vi "7HP.vi"() -> (0 "DAQ Error":errorcluster)   [LabVIEW 2017]
doc: "Use this plug-in with the Nathan 7609 data acquisition system"
uses:
  7HP/ctls/Cmd (USB).ctl
  Globals/Meas_global.vi
  Globals/Extra_Commands_Global.vi
  Globals/Dynamic_call_global.ph.vi
  Globals/Trav_pos_global.vi
panel:
  # "Do not close this window between blocks"
  # "PN 18/10/2017"
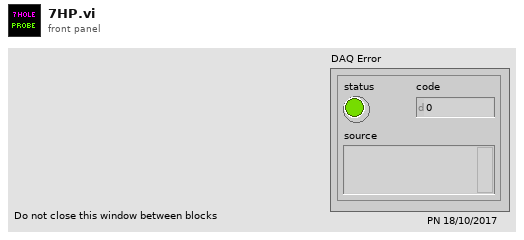
[diagram p1: front panel]
types:
  T1 = typedef "Analysis_info_cluster.ctl" = cluster{"Colour":u32, "Inst type":T2, "Inst name":string, "Symbol":string, "Code name":string, "Extra Info":string, "Inst Array":T3, "Extra Titles":string[], "Extra Values":string[], "U":dbl, "u^2":dbl, "u^3":dbl, "u^4":dbl, "Skew_u":dbl, "Kurt_u":dbl, "Sd Error in Mean":dbl, "% u'/U":dbl, "X":dbl, "Y":dbl, "Z":dbl, "Timescale integral Estimate":dbl, "Sd Error in Variance":dbl, "Calib File":path, "Calib Constants":dbl[], "Output Position":bool, "Full Stats":bool, "Av Sampling Rate":dbl, "Av No of Samples":dbl, "Total Meas Time (s)":dbl, "ADAM Ch Name":string, "Max value":dbl, "Min value":dbl, "Req Sample Rate Hz":dbl, "Sync Delay Time (s)":dbl, "Ch No":i16, "Device ID":string, "Use Latest Calib":bool, "Port":string}
  T2 = typedef "Inst_type.ctl" = enum16{"Propeller anemometer", "Raw voltage", "Pressure Transducer", "Pitot-static tube", "Preston tube", "Hot wire", "Cross wire 1", "Cross wire 2", "Generic Linear", "Generic Polynomial", "Generic BackPoly", "Fast FID", "Thermocouple", "Cold wire", "Pulsed Wire", "LDA Vel", "LDA Tran time", "LDA Arr time", "Microphone"}
  T3 = typedef "Instrument_Array.ctl" = enum16{"PWA", "LDA", "Analogue"}
  T4 = typedef "Traverse_cluster.ctl" = cluster{"Start X":sgl, "Start Y":sgl, "Start Z":sgl, "End X":sgl, "End Y":sgl, "End Z":sgl, "No. of pts.":i32, "Spacing":T5, "Filename":path, "Tunnel Speed":dbl, "Averaging time (min)":dbl, "Extra Commands":string, "Carrier_1 Q (l/min)":dbl, "Carrier_2 Q (l/min)":dbl, "Trace Gas Concentration (%)":dbl, "Specific Arguments":string, "Comments":string, "Row No":i32, "Row Type Selector":T6, "Completion time":string, "Row Duration (mins)":dbl, "No. of Valid pts.":i32, "Meas Setup File":string}
  T5 = typedef "Spacing.ctl" = enum16{"Linear", "Log", "Gauss", "Specified", "N/A"}
  T6 = typedef "Multi_run_mode.ctl" = enum16{"Move Traverse Only", "Set Tunnel Speed Only", "Set Source Only", "Set Measurement Conditions", "Single Measurement", "Vertical Profile", "Lateral Profile", "Longitudinal Profile", "Explore Volume", "Multi-Axis Profile", "Auto Calibrate", "Meas Fast FID Bkgnd", "Check Beam Power", "Scanning Valve Measurement", "Run VI Named:", "Set ADAM Ch", "Wait (minutes)", "Send Message", "Synchronize With:", "Fall Back to this Row", "Turn Off Row Repeating", "Blank Row", "Traverse 3D Volume"}
  T7 = typedef "Trigger_Mode.ctl" = enum16{"Free Running", "Start on Trigger", "Trigger Every Block", "Trigger Every Sample"}
  T8 = typedef "Cmd (USB).ctl" = string
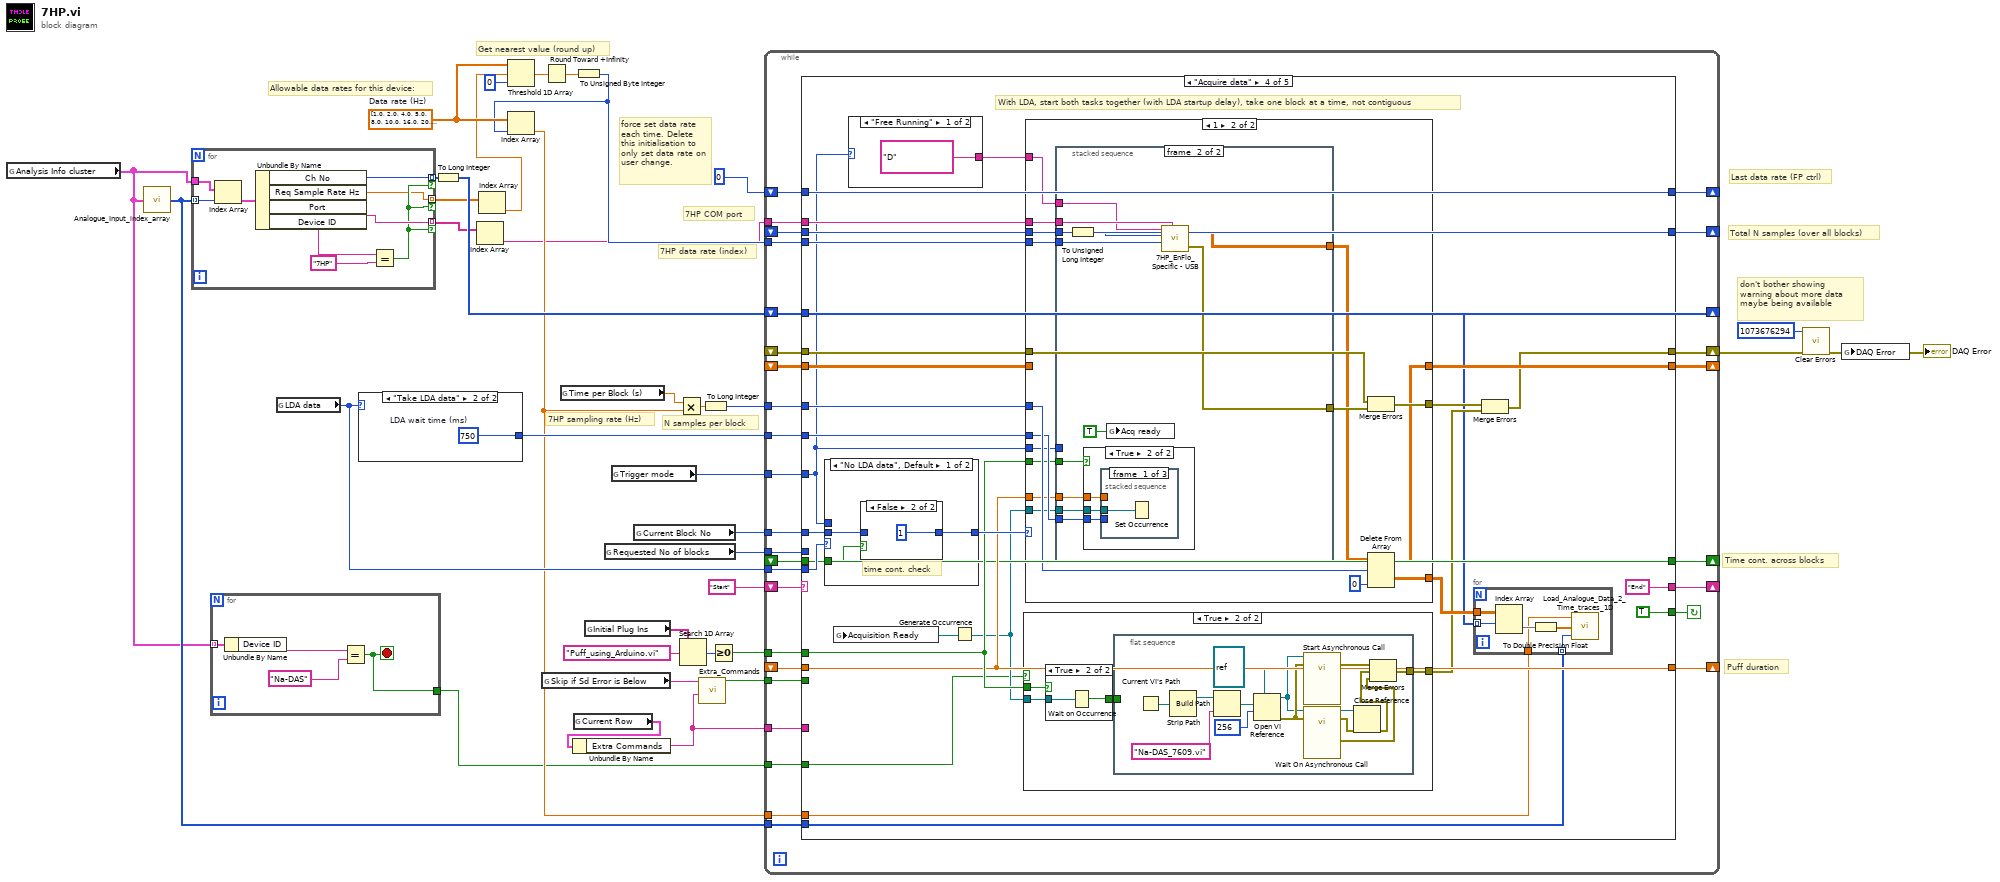
[diagram p0: block diagram]
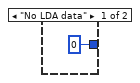
[diagram p2: hidden frame]
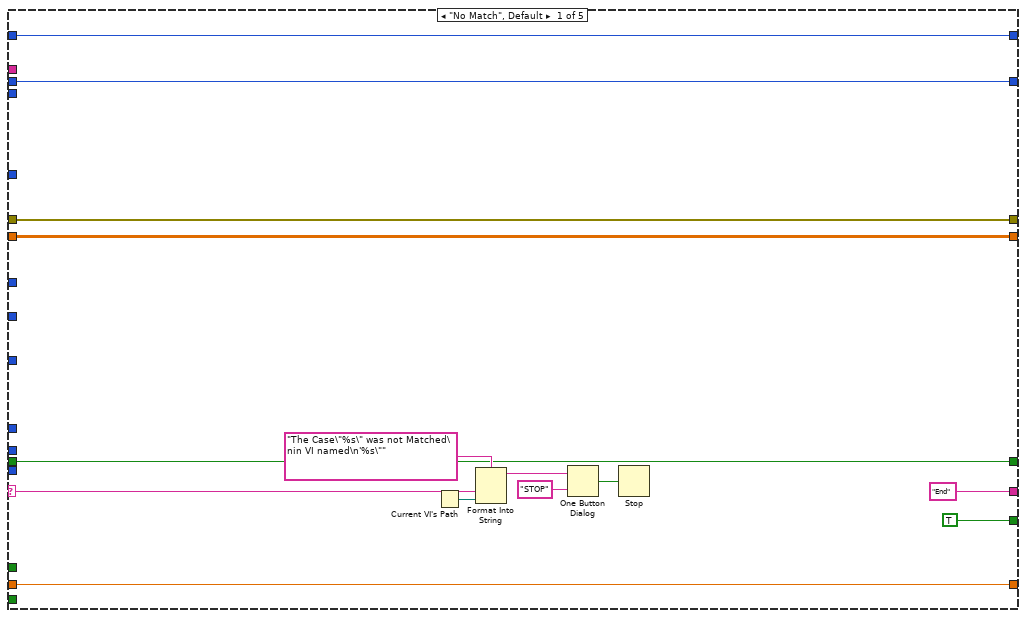
[diagram p3: hidden frame]
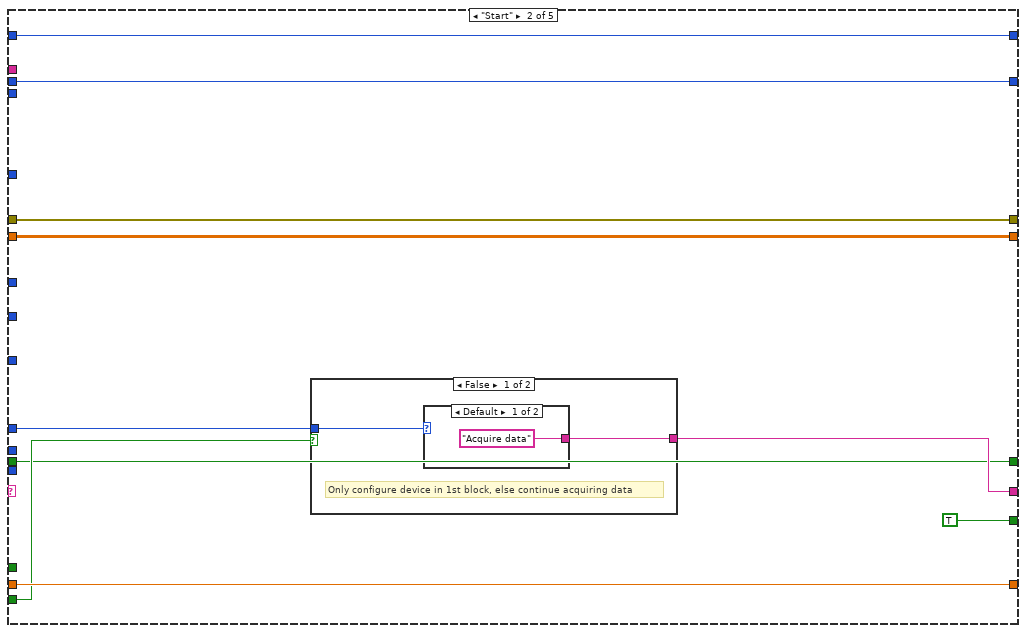
[diagram p4: hidden frame]
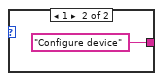
[diagram p5: hidden frame]
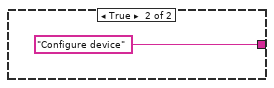
[diagram p6: hidden frame]
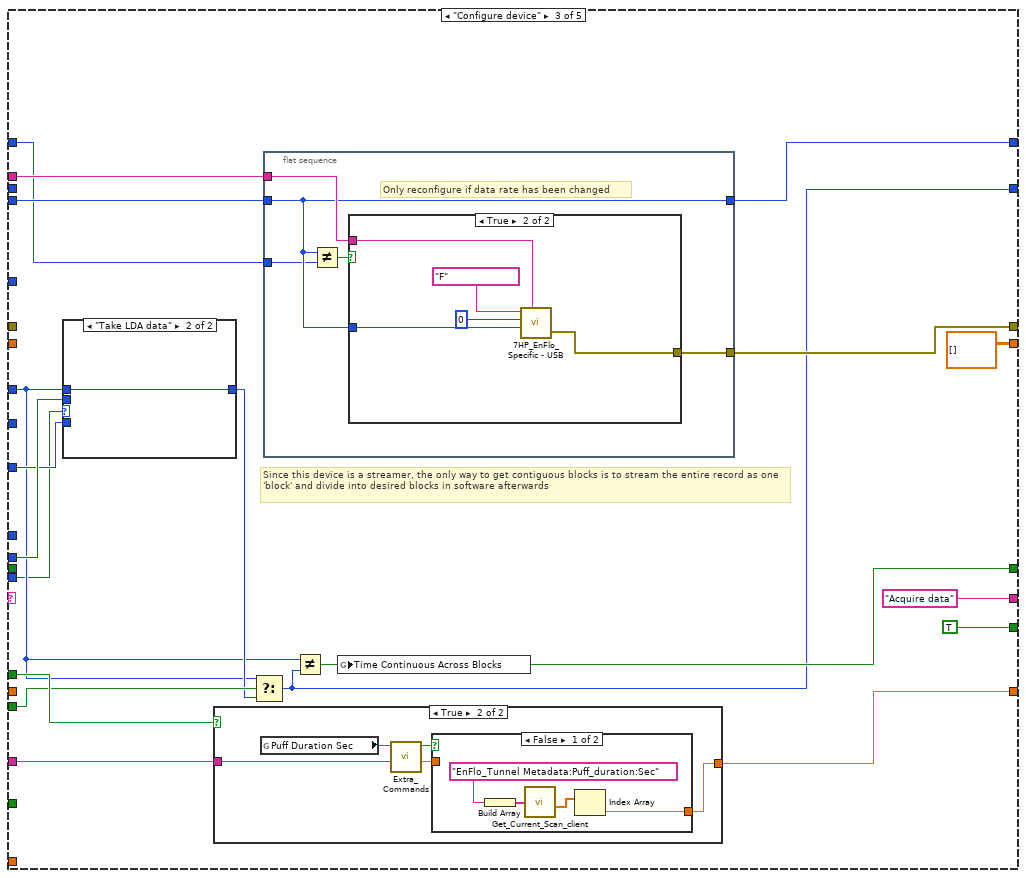
[diagram p7: hidden frame]
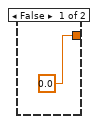
[diagram p8: hidden frame]
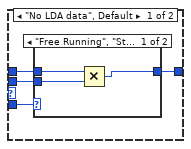
[diagram p10: hidden frame]
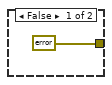
[diagram p12: hidden frame]
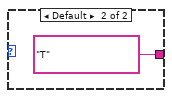
[diagram p13: hidden frame]
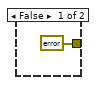
[diagram p14: hidden frame]
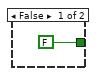
[diagram p15: hidden frame]
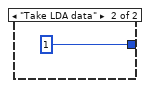
[diagram p17: hidden frame]
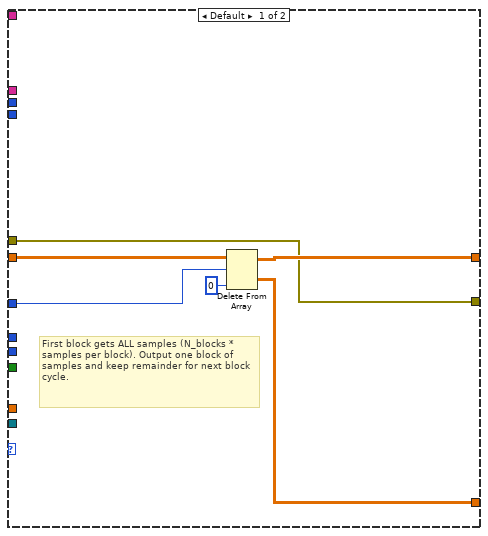
[diagram p18: hidden frame]
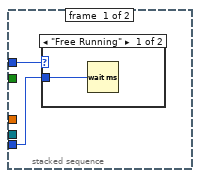
[diagram p19: hidden frame]
diagram:
  w16 = dbl[] [1.0, 2.0, 4.0, 5.0, 8.0, 10.0, 16.0, 20.0, 25.0, 32.0, 40.0, 50.0, 64.0, 80.0, 100.0, 125.0, 160.0, 200.0, 250.0, 320.0, 400.0, 500.0, 625.0, 800.0, 1000.0]  # Data rate (Hz)
  # "N samples per block"
  # "7HP sampling rate (Hz)"
  # "7HP COM port"
  # "7HP data rate (index)"
  # "Allowable data rates for this device:"
  # "Get nearest value (round up)"
  # "force set data rate each time. Delete this initialisation to only set data rate on user change."
  # "Last data rate (FP ctrl)"
  # "Total N samples (over all blocks)"
  # "don't bother showing warning about more data maybe being available"
  # "Time cont. across blocks"
  # "Puff duration"
  n1 = global read "Meas_global.vi" "Analysis Info cluster"() -> (w2:T1[])
  n2 = call "Analogue_Input_index_array.vi"("Analysis Info cluster"=w2) -> ("Array"=w9:i32[])
  n3 = for {
    tunnel: [w45] -> w14 mode=indexing if=w38
    tunnel: [w37] -> w3 mode=indexing if=w38
    tunnel: w2 -> [w44]
    tunnel: w9 -> [w43] mode=indexing
    tunnel: [w41] -> w6 mode=indexing if=w38
    n4 = Index Array(array=w44, index=w43) -> (element=w42:T1)
    n5 = Unbundle By Name(w42) -> ("Ch No"=w45:i16, "Req Sample Rate Hz"=w37:dbl, "Port"=w41:string, "Device ID"=w40:string)
    n6 = Equal?(x=w40, y="7HP" ("Device ID")) -> (x = y?=w38:bool)
  }
  n7 = for {
    tunnel: w2 -> [w47] mode=indexing
    tunnel: [w46] -> w1
    stop <- w46 stop-if-true
    n8 = Unbundle By Name(w47) -> ("Device ID"=w49:string)
    n9 = Equal?(x=w49, y="Na-DAS" ("Device ID")) -> (x = y?=w46:bool)
  }
  n10 = global read "Meas_global.vi" "LDA data"() -> (w33:enum16{"No LDA data", "Take LDA data"})
  n11 = case shown="\"Take LDA data\"" w33 {
    tunnel: [u32 0 ("LDA wait time (ms)") w51] -> w28
    frame "No LDA data" {
    }
    frame "Take LDA data" {
      w51 = u32 750  # LDA wait time (ms)
    }
  }
  n12 = To Long Integer(number=w14) -> (32bit integer=w13:i32[])
  n13 = Index Array(array=w6) -> (element=w5:string)  [unwired: 1 in]
  n14 = Index Array(array=w3) -> (element=w4:dbl)  [unwired: 1 in]
  n15 = Threshold 1D Array(1:0 ("start index (0)"), 2:w4, 3:w16) -> (0:w17:dbl)
  n16 = global read "Extra_Commands_Global.vi" "Skip if Sd Error is Below"() -> (w25:string)
  n17 = Round Toward +Infinity(x=w17) -> (ceil(x): smallest int >= x=w15:dbl)
  n18 = global read "Meas_global.vi" "Time per Block (s)"() -> (w12:dbl)
  n19 = global read "Trav_pos_global.vi" "Current Row"() -> (w26:T4)
  n20 = Unbundle By Name(w26) -> ("Extra Commands"=w24:string)
  n21 = To Unsigned Byte Integer(number=w15) -> (unsigned 8bit integer=w7:u8)
  n22 = Index Array(array=w16, index=w7) -> (element=w8:dbl)
  n23 = global read "Dynamic_call_global.ph.vi" "Initial Plug Ins"() -> (w30:string[])
  n24 = global read "Meas_global.vi" "Requested No of blocks"() -> (w27:i32)
  n25 = global read "Meas_global.vi" "Trigger mode"() -> (w35:T7)
  n26 = global read "Meas_global.vi" "Current Block No"() -> (w34:i32)
  n27 = Multiply(x=w12, y=w8) -> (x*y=w11:dbl)
  n28 = Search 1D Array(1D array=w30, element="Puff_using_Arduino.vi") -> (index of element=w32:i32)  [unwired: 1 in]
  n29 = call "Extra_Commands.vi"("String to Search"=w24, "Command"=w25) -> ("Command Found"=w23:bool)  [unwired: 2 in, 3 out]
  n30 = To Long Integer(number=w11) -> (32bit integer=w10:i32)
  n31 = Greater Or Equal To 0?(x=w32) -> (x >= 0?=w29:bool)
  n32 = while {
    shift-left: "Start" -> [w81]
    shift-right: [w70] -> _
    tunnel: w10 -> [w80]
    tunnel: w34 -> [w79]
    tunnel: w35 -> [w77]
    tunnel: w33 -> [w76]
    tunnel: w27 -> [w75]
    shift-right: [w73] -> w20
    shift-left: _ -> [w74]
    shift-right: [w72] -> _
    shift-left: _ -> [w71]
    tunnel: w28 -> [w69]
    tunnel: w29 -> [w68]
    shift-right: [w67] -> _
    shift-left: _ -> [w66]
    shift-right: [w65] -> _
    shift-left: w13 -> [w65]
    tunnel: w24 -> [w64]
    tunnel: w23 -> [w63]
    shift-right: [w62] -> _
    shift-left: _ -> [w61]
    tunnel: w5 -> [w60]
    tunnel: w7 -> [w59]
    shift-right: [w58] -> _
    shift-left: _ -> [w57]
    shift-right: [w56] -> _
    shift-left: u8 0 ("Pressure data rate (Hz)") -> [w55]
    tunnel: w9 -> [w54]
    tunnel: w8 -> [w53]
    tunnel: w1 -> [w52]
    stop <- w78 continue-if-true
    n33 = case shown="\"Acquire data\"" w81 {
      selector: w81 -> [w88 _ _ _ _]
      tunnel: ["End" w102 "Acquire data" ("f") "End" "End" ("f")] -> w70
      tunnel: w80 -> [_ _ w118 w172 _]
      tunnel: w79 -> [_ w103 _ w182 _]
      tunnel: [TRUE TRUE TRUE TRUE FALSE] -> w78
      tunnel: w77 -> [_ _ w124 w162 _]
      tunnel: w76 -> [_ _ w116 w180 _]
      tunnel: w75 -> [_ _ w128 _ _]
      tunnel: w74 -> [w87 w104 _ w186 w272]
      tunnel: [w87 w104 w127 w173 w272] -> w73
      tunnel: [w86 w101 sgl[][] [] ("Channel volts") w184 w275] -> w72
      tunnel: w71 -> [w86 w101 _ w185 w275]
      tunnel: w69 -> [_ _ _ w181 _]
      tunnel: w68 -> [_ _ w123 w179 _]
      tunnel: [w85 w100 w122 w178 w274] -> w67
      tunnel: w66 -> [w85 w100 _ w178 w274]
      tunnel: w65 -> [_ _ _ w166 _]
      tunnel: w64 -> [_ _ w121 _ _]
      tunnel: w63 -> [_ w99 w120 _ _]
      tunnel: [w84 w98 w117 w176 w273] -> w62
      tunnel: w61 -> [w84 w98 _ w176 w273]
      tunnel: w60 -> [_ _ w115 w170 _]
      tunnel: w59 -> [_ _ w114 w169 _]
      tunnel: [w82 w96 w113 w167 w270] -> w58
      tunnel: w57 -> [w82 w96 _ w167 w270]
      tunnel: [w83 w97 w112 w168 w271] -> w56
      tunnel: w55 -> [w83 w97 w111 w168 w271]
      tunnel: w54 -> [_ _ _ w165 _]
      tunnel: w53 -> [_ _ _ w164 _]
      tunnel: w52 -> [_ _ _ w161 _]
      frame "No Match", Default {
        n34 = Current VI's Path() -> (path=w91:path)
        n35 = Format Into String(format string="The Case\"%s\" was not Matched\nin VI named\n'%s\"" ("Format String"), w88, w91) -> (resulting string=w94:string)  [unwired: 2 in, 1 out]
        n36 = One Button Dialog(message=w94, button name ("OK")="STOP") -> (true=w92:bool)
        n37 = Stop(stop? (T)=w92) -> ()
      }
      frame "Start" {
        n38 = case shown="False" w99 {
          tunnel: w103 -> [w107 _]
          tunnel: [w106 "Configure device" ("f")] -> w102
          frame False {
            # "Only configure device in 1st block, else continue acquiring data"
            n39 = case shown="Default" w107 {
              tunnel: ["Acquire data" ("f") "Configure device" ("f")] -> w106
              frame Default {
              }
              frame 1 {
              }
            }
          }
          frame True {
          }
        }
      }
      frame "Configure device" {
        # "Since this device is a streamer, the only way to get contiguous blocks is to stream the entire record as one 'block' and divide into desired blocks in software afterwards"
        n40 = case shown="\"Take LDA data\"" w116 {
          tunnel: [w142 w149] -> w119
          tunnel: w118 -> [w144 w149]
          tunnel: w128 -> [w143 _]
          tunnel: w124 -> [w141 _]
          frame "No LDA data", Default {
            n41 = case shown="\"Free Running\", \"Start on Trigger\"" w141 {
              tunnel: w144 -> [w147 w148]
              tunnel: w143 -> [w146 _]
              tunnel: [w145 w148] -> w142
              frame "Free Running", "Start on Trigger" {
                n42 = Multiply(x=w147, y=w146) -> (x*y=w145:i32)
              }
              frame "Trigger Every Block", Default {
              }
            }
          }
          frame "Take LDA data" {
          }
        }
        n43 = case shown="True" w123 {
          tunnel: [0.0 w135] -> w122
          tunnel: w121 -> [_ w131]
          frame False {
          }
          frame True {
            n44 = global read "Extra_Commands_Global.vi" "Puff Duration Sec"() -> (w134:string)
            n45 = call "Extra_Commands.vi"("String to Search"=w131, "Command"=w134) -> ("Numeric Value"=w132:dbl, "Command Found"=w133:bool)  [unwired: 2 in, 2 out]
            n46 = case shown="False" w133 {
              tunnel: [w136 w140] -> w135
              tunnel: w132 -> [_ w140]
              frame False {
                n47 = Build Array("EnFlo_Tunnel Metadata:Puff_duration:Sec") -> (w138:string[])
                n48 = call "Get_Current_Scan_client.vi"("ADAM Ch Names"=w138) -> ("Numerical Values"=w139:dbl[])  [unwired: 1 in, 2 out]
                n49 = Index Array(array=w139) -> (element=w136:dbl)  [unwired: 1 in]
              }
              frame True {
              }
            }
          }
        }
        n50 = Select(t=w118, s=w120, f=w119) -> (s? t:f=w113:i32)
        n51 = flat-sequence {
          tunnel: [w154] -> w127
          tunnel: w115 -> [w153]
          tunnel: w114 -> [w151]
          tunnel: [w151] -> w112
          tunnel: w111 -> [w150]
          frame #0 {
            # "Only reconfigure if data rate has been changed"
            n52 = Not Equal?(x=w151, y=w150) -> (x != y?=w152:bool)
            n53 = case shown="True" w152 {
              tunnel: [errorcluster {"status"=FALSE, "code"=0, "source"=""} ("error IO") w157] -> w154
              tunnel: w153 -> [_ w156]
              tunnel: w151 -> [_ w158]
              frame False {
              }
              frame True {
                n54 = call "7HP_EnFlo_Specific - USB.vi"("COM port"=w156, "Data rate (Hz)"=w158, "N samples"=u32 0, "Command"=T8 "F") -> ("Error"=w157:errorcluster)  [unwired: 2 in, 1 out]
              }
            }
          }
        }
        n55 = Not Equal?(x=w118, y=w113) -> (x != y?=w117:bool)
        n56 = global write "Meas_global.vi" "Time Continuous Across Blocks"(w117) -> ()
      }
      frame "Acquire data" {
        # "With LDA, start both tasks together (with LDA startup delay), take one block at a time, not contiguous"
        n57 = case shown="\"No LDA data\", Default" w180 {
          tunnel: w182 -> [w220 _]
          tunnel: w162 -> [_ _]
          tunnel: [w221 1 ("Current Block No")] -> w183
          tunnel: w176 -> [w219 _]
          frame "No LDA data", Default {
            # "time cont. check"
            n58 = case shown="False" w219 {
              tunnel: [w222 1 ("Current Block No")] -> w221
              tunnel: w220 -> [w222 _]
              frame True {
              }
              frame False {
              }
            }
          }
          frame "Take LDA data" {
          }
        }
        n59 = case shown="\"Free Running\"" w162 {
          tunnel: [T8 "D" ("Command") T8 "T" ("Command")] -> w163
          frame "Free Running" {
          }
          frame Default {
          }
        }
        n60 = Generate Occurrence() -> (w171:refnum<k4>)
        n61 = global write "Meas_global.vi" "Acquisition Ready"(w171) -> ()
        n62 = case shown="True" w161 {
          tunnel: w179 -> [_ w198]
          tunnel: w171 -> [_ w200]
          tunnel: [errorcluster {"status"=FALSE, "code"=0, "source"=""} ("error IO") w199] -> w174
          frame False {
          }
          frame True {
            n63 = case shown="True" w198 {
              tunnel: [FALSE ("timed out") w204] -> w201
              tunnel: w200 -> [_ w203]
              frame False {
              }
              frame True {
                n64 = Wait on Occurrence(2:w203) -> (0:w204:bool)  [unwired: 2 in]
              }
            }
            n65 = flat-sequence {
              tunnel: w201 -> [_]
              tunnel: [w206] -> w199
              frame #0 {
                n66 = Current VI's Path() -> (path=w216:path)
                n67 = Strip Path(path=w216) -> (stripped path=w215:path)  [unwired: 1 out]
                n68 = Build Path(base path=w215, name or relative path="Na-DAS_7609.vi") -> (appended path=w217:path)
                n69 = Open VI Reference(type specifier VI Refnum (for type only)=refnum<vi> refnum, vi path=w217, options=256) -> (vi reference=w211:refnum<vi>, error out=w212:errorcluster)  [unwired: 3 in]
                n70 = call-by-ref "Start Asynchronous Call"(reference=w211, error in=w212) -> (error out=w208:errorcluster)  [unwired: 1 in, 2 out]
                n71 = call-by-ref "Wait On Asynchronous Call"(reference=w211, error in=w212) -> (reference out=w210:refnum<vi>, error out=w209:errorcluster, 0:"error out"=w205:errorcluster)  [unwired: 1 in]
                n72 = Close Reference(reference=w210, error in (no error)=w209) -> (error out=w207:errorcluster)
                n73 = Merge Errors(w208, w207, w205) -> (w206:errorcluster)
              }
            }
          }
        }
        n74 = case shown="1" w183 {
          tunnel: w186 -> [w226 w246]
          tunnel: [w226 w245] -> w175
          tunnel: [w228 w242] -> w184
          tunnel: w172 -> [w227 w243]
          tunnel: w185 -> [w229 _]
          tunnel: [w225 w240] -> w177
          tunnel: w181 -> [_ w239]
          tunnel: w171 -> [_ w238]
          tunnel: w179 -> [_ w237]
          tunnel: w178 -> [_ w236]
          tunnel: w162 -> [_ w235]
          tunnel: w170 -> [_ w234]
          tunnel: w169 -> [_ w233]
          tunnel: w167 -> [_ w232]
          tunnel: w163 -> [_ w231]
          frame Default {
            # "First block gets ALL samples (N_blocks * samples per block). Output one block of samples and keep remainder for next block cycle."
            n75 = Delete From Array(array=w229, length=w227, index (col)=0 ("disabled index (col)")) -> (deleted portion=w225:sgl[][], array with subset deleted=w228:sgl[][])  [unwired: 1 in]
          }
          frame 1 {
            n76 = stacked-sequence {
              tunnel: [_ w252] -> w244
              tunnel: [_ w253] -> w247
              tunnel: w238 -> [_ w261]
              tunnel: w239 -> [w249 w260]
              tunnel: w237 -> [_ w259]
              tunnel: w236 -> [_ w258]
              tunnel: w235 -> [w248 _]
              tunnel: w234 -> [_ w256]
              tunnel: w233 -> [_ w255]
              tunnel: w232 -> [_ w254]
              tunnel: w231 -> [_ w251]
              frame #0 {
                n77 = case shown="\"Free Running\"" w248 {
                  tunnel: w249 -> [w250 _]
                  frame "Free Running" {
                    n78 = Wait (ms)(milliseconds to wait=w250) -> ()  [unwired: 1 out]
                  }
                  frame Default {
                  }
                }
              }
              frame #1 {
                n79 = To Unsigned Long Integer(number=w254) -> (unsigned 32bit integer=w257:u32)
                n80 = case shown="True" w259 {
                  tunnel: w261 -> [w263 w266]
                  tunnel: w258 -> [_ w265]
                  tunnel: w260 -> [_ w264]
                  frame False {
                    n81 = Set Occurrence(w263) -> ()
                  }
                  frame True {
                    n82 = stacked-sequence {
                      tunnel: w266 -> [w267 _ _]
                      tunnel: w265 -> [_ _ w269]
                      tunnel: w264 -> [_ w268 _]
                      frame #0 {
                        n83 = Set Occurrence(w267) -> ()
                      }
                      frame #1 {
                        n84 = Wait (ms)(milliseconds to wait=w268) -> ()  [unwired: 1 out]
                      }
                      frame #2 {
                        n85 = call "Puff_using_Arduino_oneshot.vi"("Puff_duration:Sec"=w269) -> ()  [unwired: 7 in]
                      }
                    }
                  }
                }
                n86 = global write "Meas_global.vi" "Acq ready"(TRUE ("Acq ready")) -> ()
                n87 = call "7HP_EnFlo_Specific - USB.vi"("COM port"=w256, "Data rate (Hz)"=w255, "N samples"=w257, "Command"=w251) -> ("Error"=w253:errorcluster, "All samples out"=w252:sgl[][])  [unwired: 2 in]
              }
            }
            n88 = Merge Errors(w246, w247) -> (w245:errorcluster)
            n89 = Delete From Array(array=w244, length=w243, index (col)=0 ("disabled index (col)")) -> (deleted portion=w240:sgl[][], array with subset deleted=w242:sgl[][])  [unwired: 1 in]
          }
        }
        n90 = for {
          tunnel: w166 -> [w195] mode=indexing
          tunnel: w177 -> [w196]
          tunnel: w165 -> [w192] mode=indexing
          tunnel: w164 -> [w191]
          n91 = Index Array(array=w196, index (row)=w195) -> (element=w194:sgl[])  [unwired: 1 in]
          n92 = To Double Precision Float(number=w194) -> (double precision float=w193:dbl[])
          n93 = call "Load_Analogue_Data_2_Time_traces_1D.vi"("Ch Index"=w192, "Voltage Array"=w193, "Sampling Rate (Hz)"=w191) -> ()  [unwired: 2 in]
        }
        n94 = Merge Errors(w175, w174) -> (w173:errorcluster)
      }
      frame "End" {
        n95 = global write "Meas_global.vi" "Acq ready"(FALSE ("Acq ready")) -> ()
      }
    }
  }
  n96 = call <vilib>:"Clear Errors.vi"("error in (no error)"=w20, "specific error code to clear (0: all)"=1073676294) -> ("error out"=w22:errorcluster)  [unwired: 4 in, 1 out]
  "DAQ Error" <- w22
  n97 = global write "Meas_global.vi" "DAQ Error"(w22) -> ()
